vi "Event Handler.vi"(8 "error in":errorcluster, 10 "Stop Event Handler":refnum<user-event>, 11 "ScrollZoomGraphChart in":refnum<class "ScrollZoomGraphChart.lvclass">) -> (0 "error out":errorcluster)   [LabVIEW 2021, in "ScrollZoomGraphChart.lvclass"]
doc: "The <b>Event Handler VI</b> is a dynamic dispatch VI that should be overwritten if events are needed to create the enhanced QControl. \n\nBy inheriting from the main Control.lvclass the overwritten <b>Event Handler VI</b> will be launched asynchronously in the initialization of the QControl.\n<b> </b> <b> </b>\n©2016 Q Software Innovations, LLC (QSI)\nwritten by Quentin Alldredge\nproduced in LabVIEW 2015\n\nsupport@qsoftwareinnovations.com\nwww.qsoftwareinnovations.com\n\nAll rights reserved.\n\nRedistribution and use in source and binary forms, with or without modification, are permitted provided that the following conditions are met:\n\n * Redistributions of source code must retain the above copyright notice, this list of conditions and the following disclaimer.\n * Redistributions in binary form must reproduce the above copyright notice, this list of conditions and the following disclaimer in the documentation and/or other materials provided with the distribution.\n * Neither the name of Q Software Innovations, LLC. nor the names of its contributors may be used to endorse or promote products derived from this software without specific prior written permission.\n\nTHIS SOFTWARE IS PROVIDED BY THE COPYRIGHT HOLDERS AND CONTRIBUTORS \"AS IS\" AND ANY EXPRESS OR IMPLIED WARRANTIES, INCLUDING, BUT NOT LIMITED TO, THE IMPLIED WARRANTIES OF MERCHANTABILITY AND FITNESS FOR A PARTICULAR PURPOSE ARE DISCLAIMED. IN NO EVENT SHALL THE COPYRIGHT OWNER OR CONTRIBUTORS BE LIABLE FOR ANY DIRECT, INDIRECT, INCIDENTAL, SPECIAL, EXEMPLARY, OR CONSEQUENTIAL DAMAGES (INCLUDING, BUT NOT LIMITED TO, PROCUREMENT OF SUBSTITUTE GOODS OR SERVICES; LOSS OF USE, DATA, OR PROFITS; OR BUSINESS INTERRUPTION) HOWEVER CAUSED AND ON ANY THEORY OF LIABILITY, WHETHER IN CONTRACT, STRICT LIABILITY, OR TORT (INCLUDING NEGLIGENCE OR OTHERWISE) ARISING IN ANY WAY OUT OF THE USE OF THIS SOFTWARE, EVEN IF ADVISED OF THE POSSIBILITY OF SUCH DAMAGE."
uses:
  ScrollZoomGraphChart.lvclass
  ScrollZoomGraphChart.lvclass/ScrollZoomGraphChart.ctl
  <vilib>/Analysis/geometry.llb/Point in Polygon Position.ctl
  <vilib>/Analysis/NI_AAL_Geometry.lvlib
  c12e3cb6-15a2-4a40-9144-b1003a9e759b.vi
  c19ac079-acbd-42d5-82d2-a79b3126a602.vi
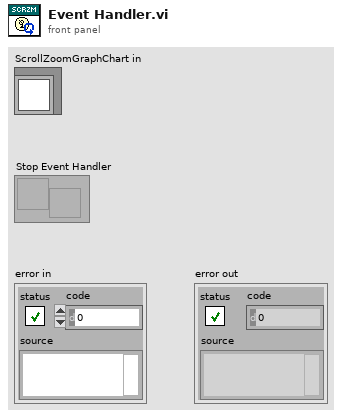
[diagram p1: front panel]
types:
  T1 = typedef "ScrollZoomGraphChart.lvclass/State Data.ctl" = cluster{"X Scales":refnum<vi>[], "Y Scales":refnum<vi>[], "Owning VI":refnum<vi>}
  T2 = typedef "NI_AAL_Geometry.lvlib/Point in Polygon Position.ctl" = u16
  T3 = typedef "LVPoint32TypeDef.ctl" = cluster{"Horizontal":i32, "Vertical":i32}
  T4 = cluster{"Shift":bool, "Ctrl":bool, "Alt":bool, "Cmd":bool, "Opt":bool}
  T5 = typedef "LVRectTypeDef.ctl" = cluster{"Left":i16, "Top":i16, "Right":i16, "Bottom":i16}
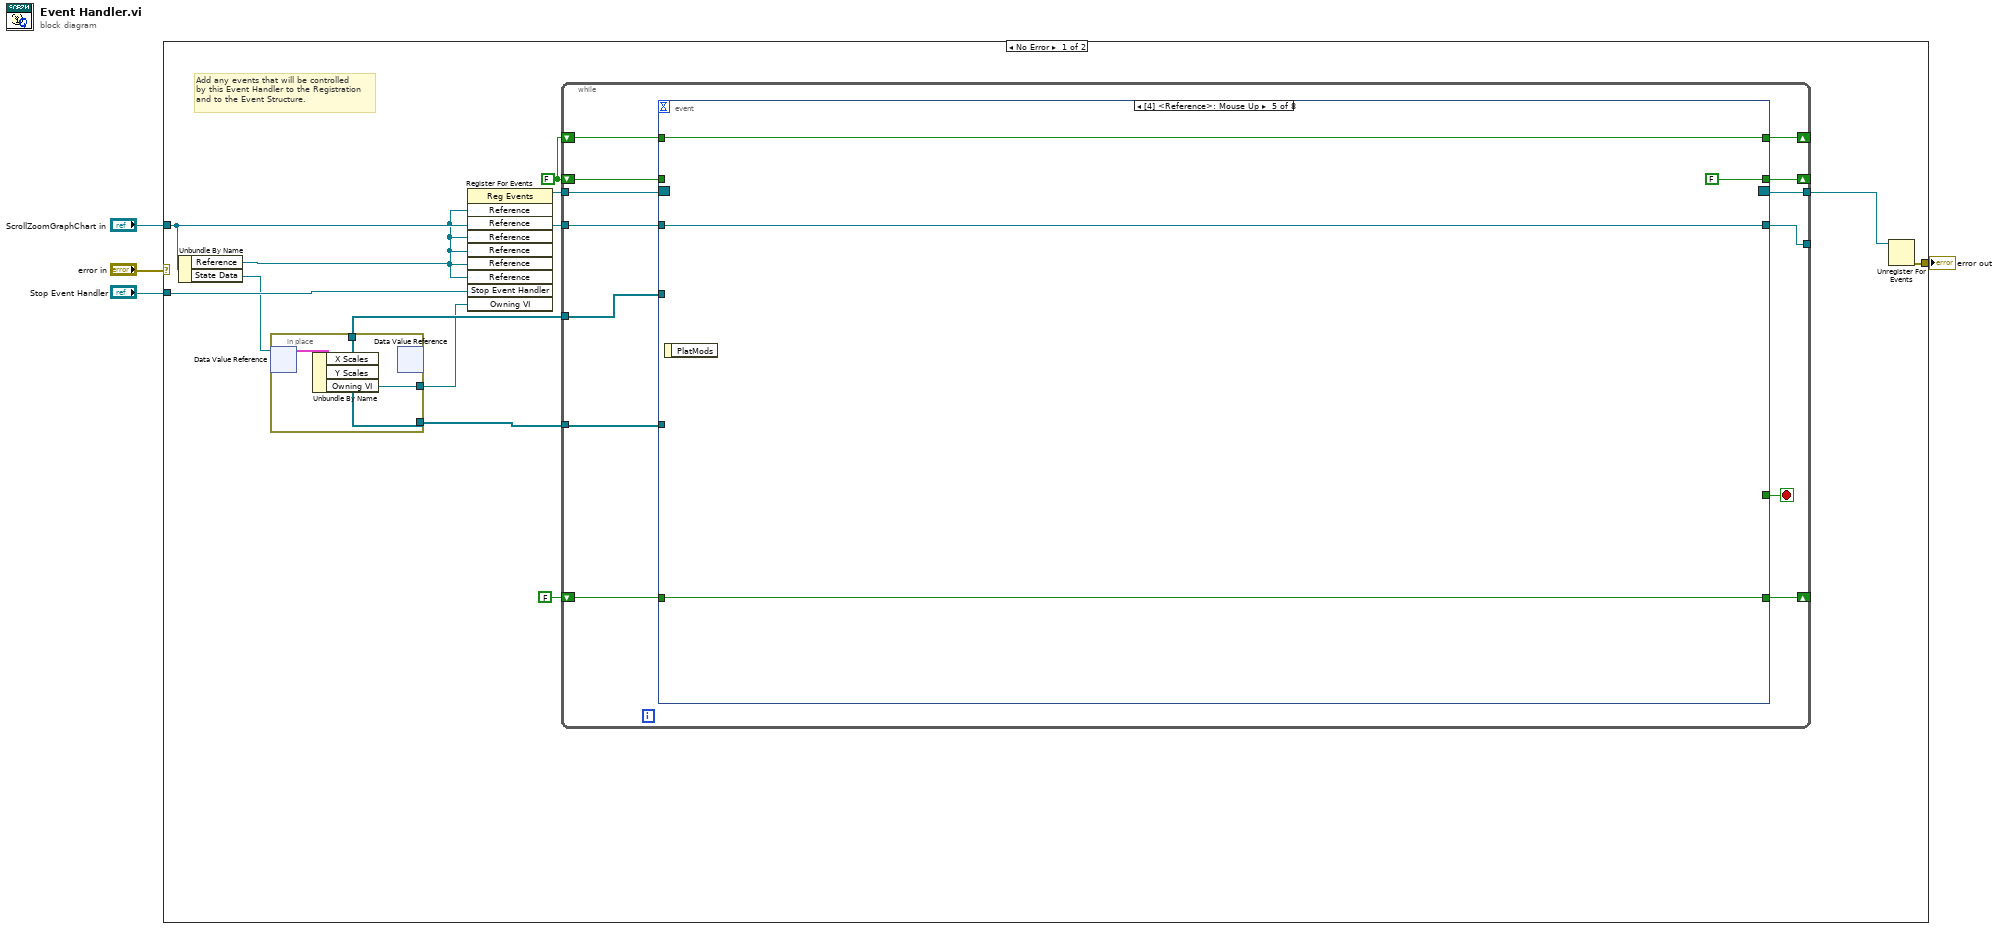
[diagram p0: block diagram]
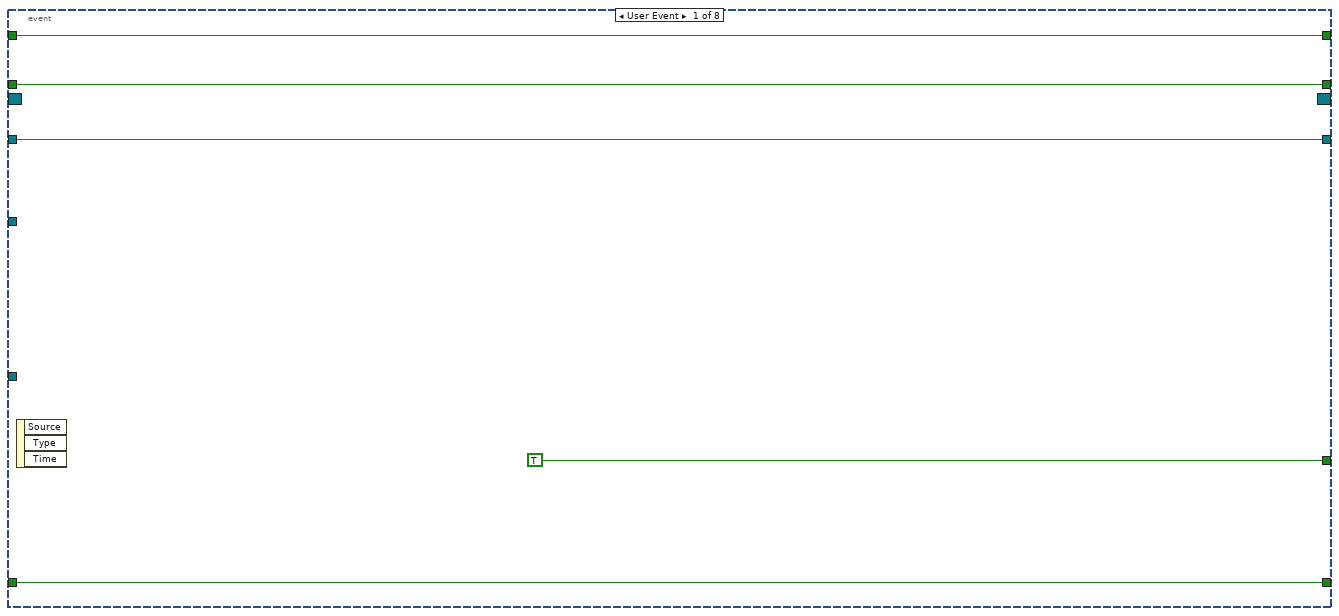
[diagram p2: hidden frame]
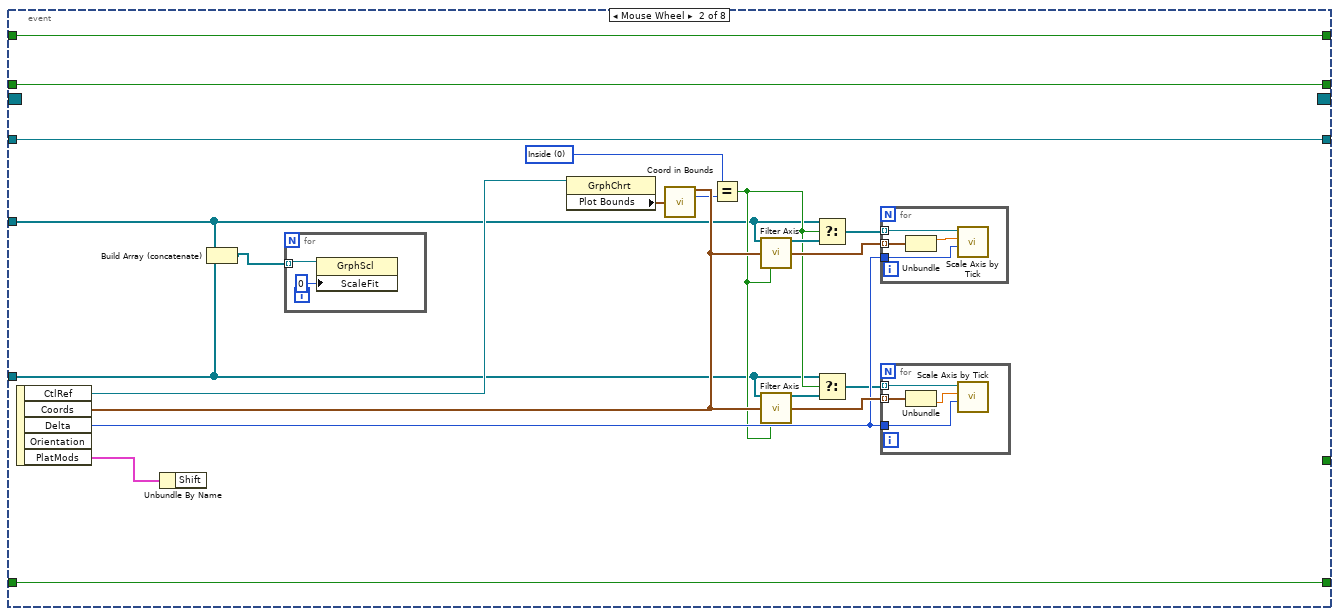
[diagram p3: hidden frame]
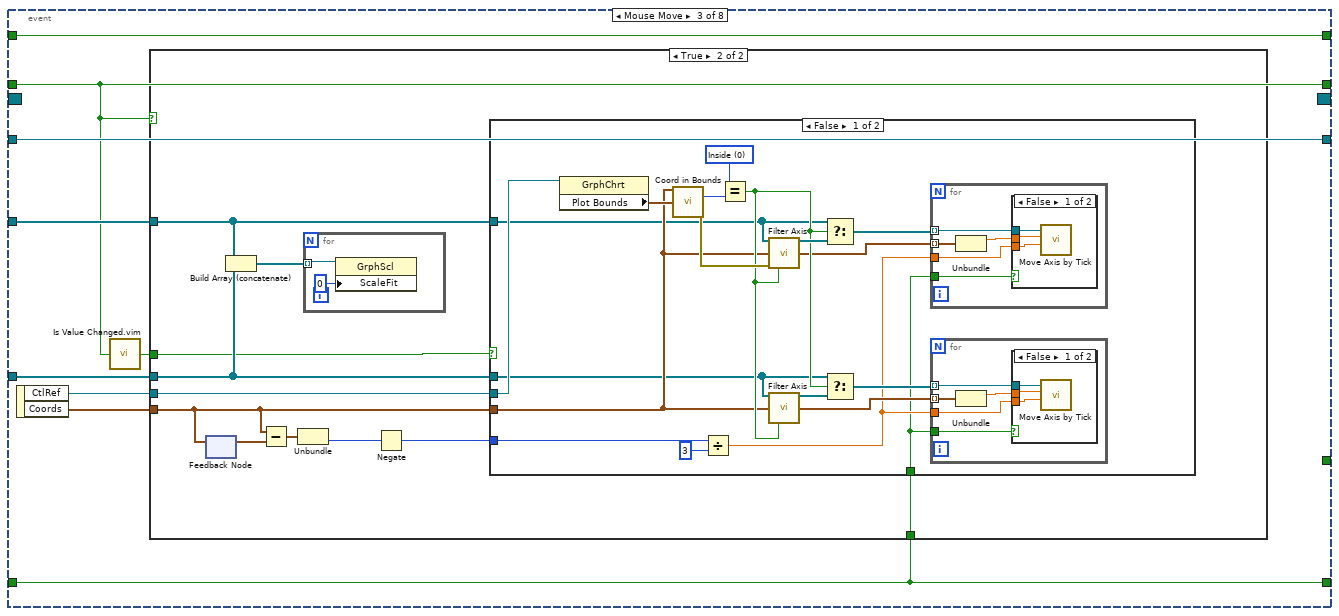
[diagram p4: hidden frame]
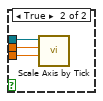
[diagram p6: hidden frame]
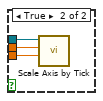
[diagram p7: hidden frame]
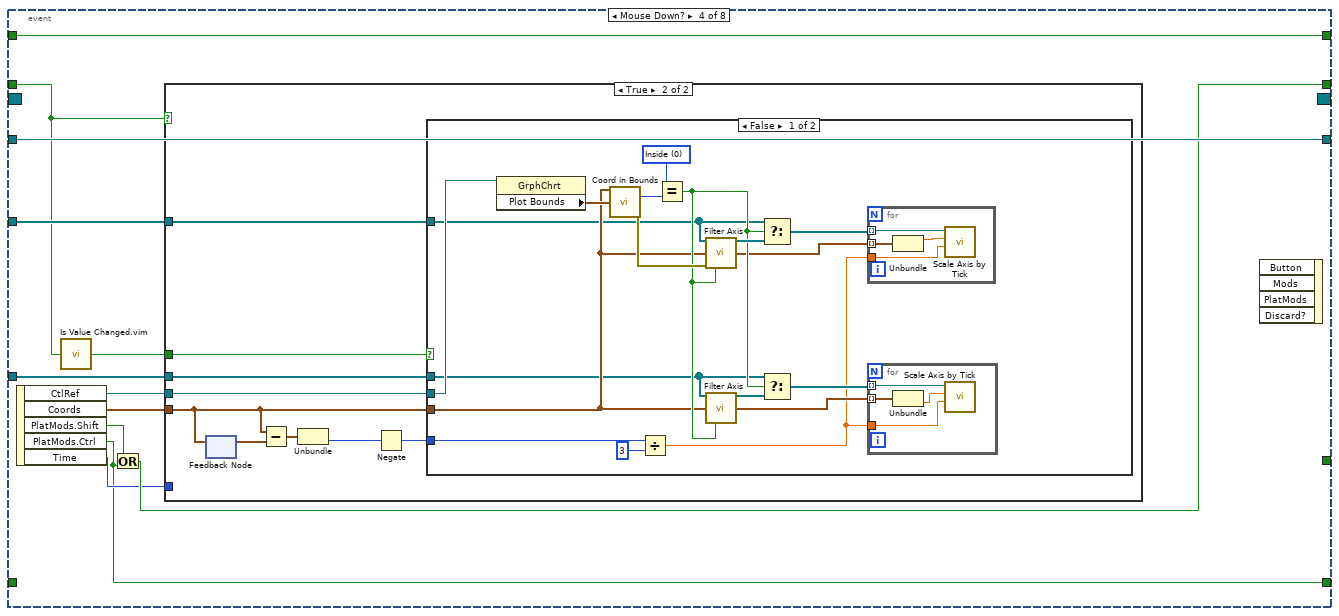
[diagram p9: hidden frame]
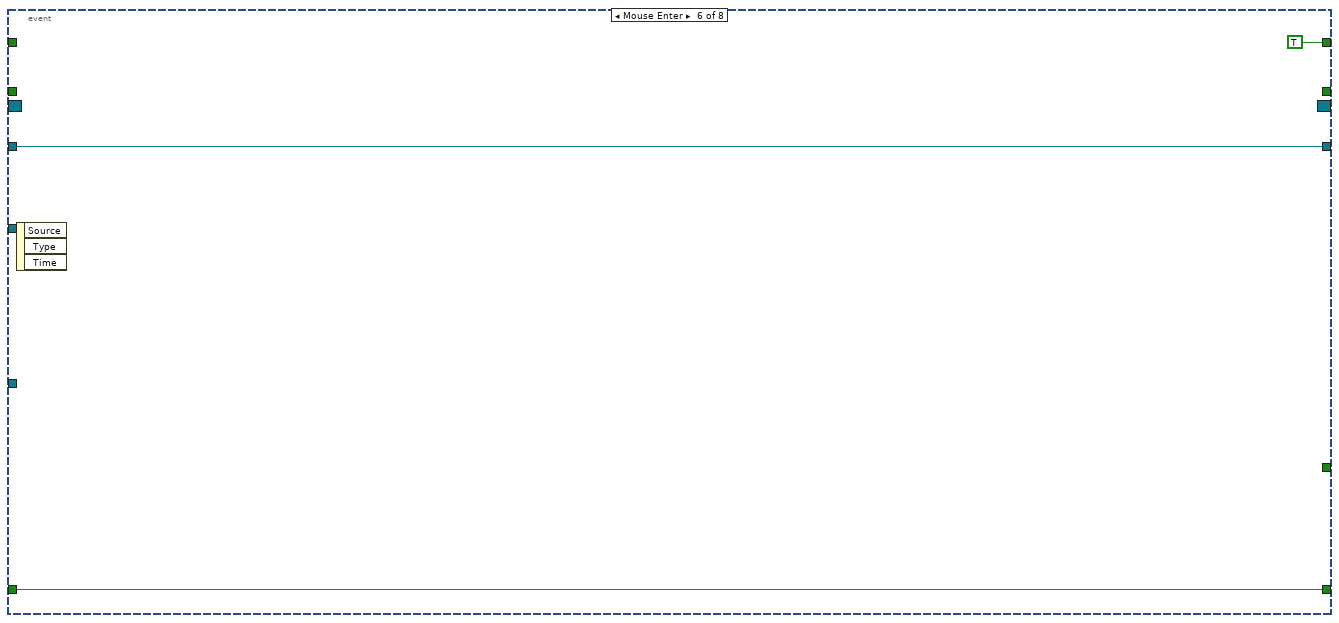
[diagram p12: hidden frame]
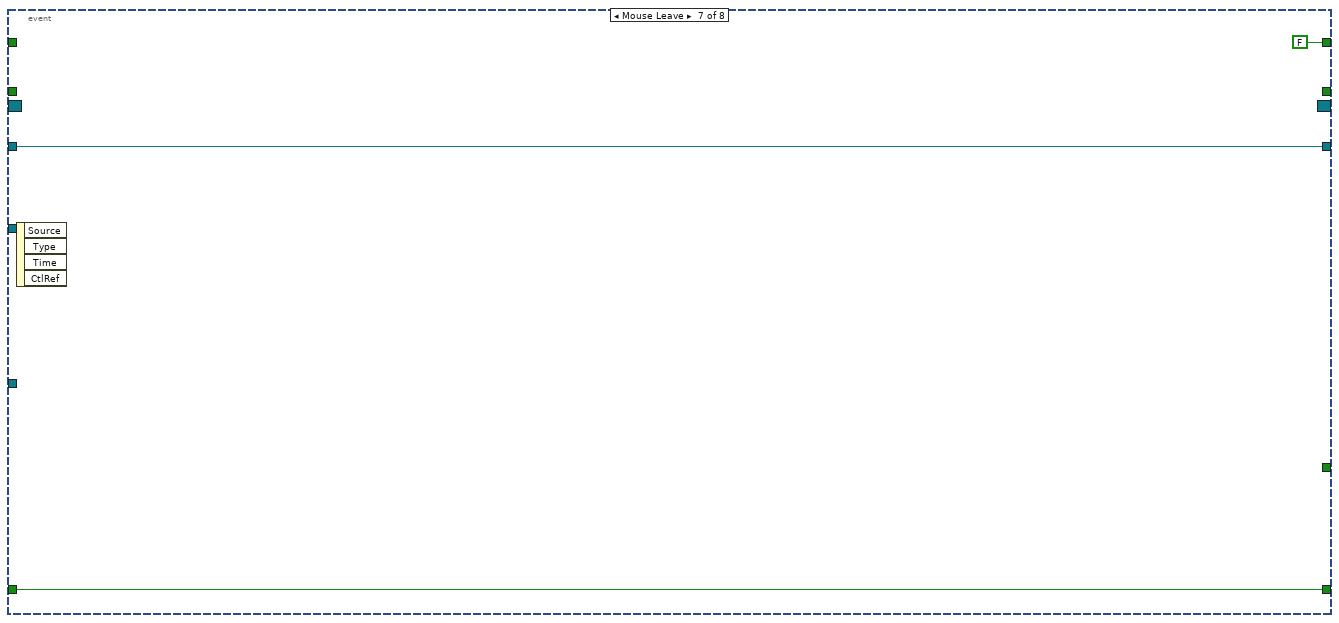
[diagram p13: hidden frame]
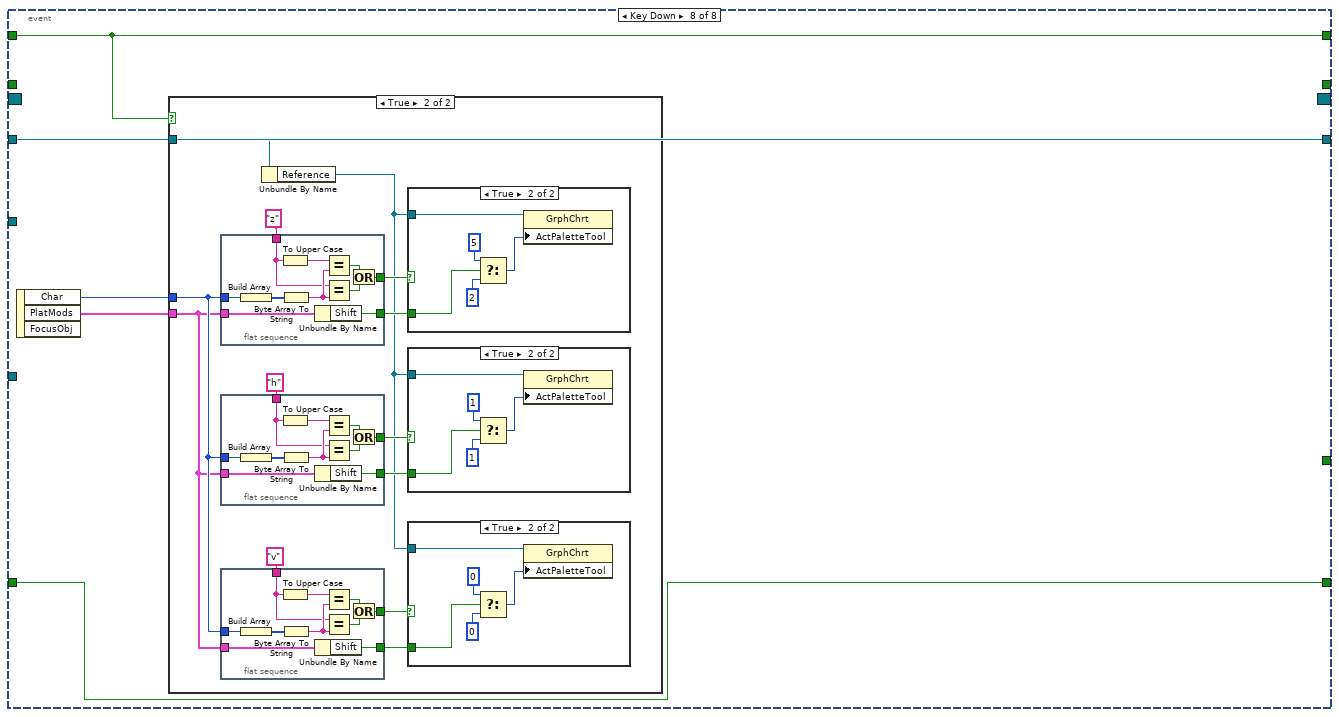
[diagram p14: hidden frame]
diagram:
  n1 = case shown="No Error" "error in" {
    selector: "error in" -> [_ w253]
    tunnel: [w16 w253] -> w3
    tunnel: "ScrollZoomGraphChart in" -> [w13 _]
    tunnel: "Stop Event Handler" -> [w15 _]
    frame No Error {
      w8 = FALSE
      # "Add any events that will be controlled\nby this Event Handler to the Registration\nand to the Event Structure."
      n2 = Unbundle By Name(w13) -> ("Reference"=w7:refnum<vi>, "State Data"=w12:refnum<data-value>)
      n3 = in-place {
        in-place-border: [w19] -> w11
        in-place-border: [w18] -> w10
        in-place-border: [w17] -> w5
        n4 = in-place-dvr #1(w12) -> (w20:T1)  [unwired: 1 out]
        n5 = Unbundle By Name(w20) -> ("X Scales"=w19:refnum<vi>[], "Y Scales"=w18:refnum<vi>[], "Owning VI"=w17:refnum<vi>)
        n6 = in-place-dvr #1() -> ()  [unwired: 1 in, 2 out]
      }
      n7 = register-events(w7, w7, w7, w7, w7, w7, w15, w5) -> (reference out=w14:refnum<event-registration>)  [unwired: 2 in, 1 out]
      n8 = while {
        tunnel: w11 -> [w32]
        tunnel: w10 -> [w31]
        tunnel: w14 -> [w30]
        tunnel: [w29] -> _
        tunnel: w13 -> [w28]
        tunnel: [w27] -> w9
        shift-right: [w26] -> _
        shift-left: w8 -> [w25]
        shift-right: [w23] -> _
        shift-left: w8 -> [w24]
        shift-right: [w22] -> _
        shift-left: FALSE ("Ctrl") -> [w21]
        stop <- w33 stop-if-true
        n9 = event shown="[4] <Reference>: Mouse Up" {
          selector: w30 -> [_ _ _ _ _ _ _ _]
          dyn-events: [_ _ _ _ _ _ _ _] -> w27
          timeout: _ -> [_ _ _ _ _ _ _ _]
          tunnel: [TRUE _ _ _ _ _ _ _] -> w33
          tunnel: w32 -> [_ w45 w77 w143 _ _ _ _]
          tunnel: w31 -> [_ w44 w76 w142 _ _ _ _]
          tunnel: [w36 w46 w78 w144 w182 w186 w189 w194] -> w29
          tunnel: w28 -> [w36 w46 w78 w144 w182 w186 w189 w194]
          tunnel: [w37 w42 w72 w138 FALSE _ _ _] -> w26
          tunnel: w25 -> [w37 w42 w72 w137 _ _ _ _]
          tunnel: w24 -> [w35 w41 w71 w135 w181 _ _ w191]
          tunnel: [w35 w41 w71 w135 w181 TRUE FALSE w191] -> w23
          tunnel: [w34 w39 w70 w133 w180 w184 w187 w190] -> w22
          tunnel: w21 -> [w34 w39 w70 _ w180 w184 w187 w190]
          event User Event {
            n10 = event-data() -> ()  [unwired: 1 in, 3 out]
          }
          event Mouse Wheel {
            w54 = T2 0 items=["Inside", "On Boundary", "Outside"] ("x")
            n11 = event-data() -> ("CtlRef"=w53:refnum<vi>, "Coords"=w56:T3, "Delta"=w50:i32, "PlatMods"=w40:T4)  [unwired: 1 in, 1 out]
            n12 = Unbundle By Name(w40) -> ()  [unwired: 1 out]
            n13 = Build Array (concatenate)(w45, w44) -> (w43:refnum<vi>[])
            n14 = for {
              tunnel: w43 -> [w61] mode=indexing
              n15 = property class="GrphScl"(reference=w61, "ScaleFit"=u8 0 ("Scale Fit")) -> ()  [unwired: 1 in, 2 out]
            }
            n16 = property class="GrphChrt"(reference=w53) -> ("Plot Bounds"=w57:T5)  [unwired: 1 in, 2 out]
            n17 = call "Coord in Bounds.vi"("Coords"=w56, "Plot Bounds"=w57) -> ("position"=w55:T2)  [unwired: 12 in, 1 out]
            n18 = Equal?(x=w54, y=w55) -> (x = y?=w47:bool)
            n19 = call "Filter Axis.vi"("Graph Scale in"=w45, "Coords"=w56, "Bypass Filter"=w47) -> ("Filter Graph Scale out"=w59:refnum<vi>[], "Axis Value"=w58:cluster{"X":dbl, "Y":dbl}[])  [unwired: 10 in, 1 out]
            n20 = call "Filter Axis.vi"("Graph Scale in"=w44, "Coords"=w56, "Bypass Filter"=w47) -> ("Filter Graph Scale out"=w52:refnum<vi>[], "Axis Value"=w51:cluster{"X":dbl, "Y":dbl}[])  [unwired: 10 in, 1 out]
            n21 = Select(t=w45, s=w47, f=w59) -> (s? t:f=w49:refnum<vi>[])
            n22 = Select(t=w44, s=w47, f=w52) -> (s? t:f=w48:refnum<vi>[])
            n23 = for {
              tunnel: w49 -> [w69] mode=indexing
              tunnel: w58 -> [w68] mode=indexing
              tunnel: w50 -> [w66]
              n24 = Unbundle(w68) -> ("X"=w67:dbl)  [unwired: 1 out]
              n25 = call "Scale Axis by Tick.vi"("Tick Scale"=w66, "Axis Focus Value"=w67, "GraphScale in"=w69) -> ()  [unwired: 9 in]
            }
            n26 = for {
              tunnel: w48 -> [w65] mode=indexing
              tunnel: w51 -> [w64] mode=indexing
              tunnel: w50 -> [w63]
              n27 = Unbundle(w64) -> ("Y"=w62:dbl)  [unwired: 1 out]
              n28 = call "Scale Axis by Tick.vi"("Tick Scale"=w63, "Axis Focus Value"=w62, "GraphScale in"=w65) -> ()  [unwired: 9 in]
            }
          }
          event Mouse Move {
            n29 = event-data() -> ("CtlRef"=w74:refnum<vi>, "Coords"=w73:T3)  [unwired: 1 in]
            n30 = call "Is Value Changed.vim"("value"=w72) -> ("changed or first call?"=w75:bool)
            n31 = case shown="True" w72 {
              tunnel: w73 -> [_ w85]
              tunnel: w74 -> [_ w89]
              tunnel: w77 -> [_ w88]
              tunnel: w76 -> [_ w87]
              tunnel: w75 -> [_ w82]
              tunnel: w70 -> [_ w79]
              frame False {
              }
              frame True {
                n32 = feedback-in #2(w85) -> ()
                n33 = feedback #2() -> (w84:T3)  [unwired: 1 in]
                n34 = Build Array (concatenate)(w88, w87) -> (w86:refnum<vi>[])
                n35 = Subtract(x=w85, y=w84) -> (x-y=w83:T3)
                n36 = Unbundle(w83) -> ("Vertical"=w81:i32)  [unwired: 1 out]
                n37 = for {
                  tunnel: w86 -> [w91] mode=indexing
                  n38 = property class="GrphScl"(reference=w91, "ScaleFit"=u8 0 ("Scale Fit")) -> ()  [unwired: 1 in, 2 out]
                }
                n39 = Negate(x=w81) -> (-x=w80:i32)
                n40 = case shown="False" w82 {
                  tunnel: w89 -> [w108 _]
                  tunnel: w88 -> [w97 _]
                  tunnel: w87 -> [w96 _]
                  tunnel: w85 -> [w101 _]
                  tunnel: w80 -> [w104 _]
                  tunnel: w79 -> [w92 _]
                  frame False {
                    w100 = T2 0 items=["Inside", "On Boundary", "Outside"] ("x")
                    n41 = property class="GrphChrt"(reference=w108) -> ("Plot Bounds"=w102:T5)  [unwired: 1 in, 2 out]
                    n42 = call "Coord in Bounds.vi"("Coords"=w101, "Plot Bounds"=w102) -> ("position"=w99:T2, "error out"=w110:errorcluster)  [unwired: 12 in]
                    n43 = Divide(x=w104, y=3) -> (x/y=w93:dbl)
                    n44 = Equal?(x=w100, y=w99) -> (x = y?=w105:bool)
                    n45 = call "Filter Axis.vi"("Graph Scale in"=w97, "Coords"=w101, "error in"=w110, "Bypass Filter"=w105) -> ("Filter Graph Scale out"=w109:refnum<vi>[], "Axis Value"=w98:cluster{"X":dbl, "Y":dbl}[])  [unwired: 9 in, 1 out]
                    n46 = call "Filter Axis.vi"("Graph Scale in"=w96, "Coords"=w101, "Bypass Filter"=w105) -> ("Filter Graph Scale out"=w107:refnum<vi>[], "Axis Value"=w94:cluster{"X":dbl, "Y":dbl}[])  [unwired: 10 in, 1 out]
                    n47 = Select(t=w97, s=w105, f=w109) -> (s? t:f=w106:refnum<vi>[])
                    n48 = Select(t=w96, s=w105, f=w107) -> (s? t:f=w95:refnum<vi>[])
                    n49 = for {
                      tunnel: w106 -> [w126] mode=indexing
                      tunnel: w98 -> [w125] mode=indexing
                      tunnel: w93 -> [w124]
                      tunnel: w92 -> [w122]
                      n50 = Unbundle(w125) -> ("X"=w123:dbl)  [unwired: 1 out]
                      n51 = case shown="False" w122 {
                        tunnel: w126 -> [w129 w132]
                        tunnel: w124 -> [w127 w131]
                        tunnel: w123 -> [w128 w130]
                        frame False {
                          n52 = call "Move Axis by Tick.vi"("Tick Scale"=w127, "Axis Focus Value"=w128, "GraphScale in"=w129) -> ()  [unwired: 9 in]
                        }
                        frame True {
                          n53 = call "Scale Axis by Tick.vi"("Tick Scale"=w131, "Axis Focus Value"=w130, "GraphScale in"=w132) -> ()  [unwired: 9 in]
                        }
                      }
                    }
                    n54 = for {
                      tunnel: w95 -> [w115] mode=indexing
                      tunnel: w94 -> [w114] mode=indexing
                      tunnel: w93 -> [w113]
                      tunnel: w92 -> [w111]
                      n55 = Unbundle(w114) -> ("X"=w112:dbl)  [unwired: 1 out]
                      n56 = case shown="False" w111 {
                        tunnel: w115 -> [w118 w121]
                        tunnel: w113 -> [w116 w120]
                        tunnel: w112 -> [w117 w119]
                        frame False {
                          n57 = call "Move Axis by Tick.vi"("Tick Scale"=w116, "Axis Focus Value"=w117, "GraphScale in"=w118) -> ()  [unwired: 9 in]
                        }
                        frame True {
                          n58 = call "Scale Axis by Tick.vi"("Tick Scale"=w120, "Axis Focus Value"=w119, "GraphScale in"=w121) -> ()  [unwired: 9 in]
                        }
                      }
                    }
                  }
                  frame True {
                  }
                }
              }
            }
          }
          event Mouse Down? {
            n59 = event-data() -> ("CtlRef"=w140:refnum<vi>, "Coords"=w139:T3, "PlatMods.Shift"=w136:bool, "PlatMods.Ctrl"=w133:bool, "Time"=w134:u32)  [unwired: 1 in]
            n60 = call "Is Value Changed.vim"("value"=w137) -> ("changed or first call?"=w141:bool)
            n61 = Or(x=w136, y=w133) -> (x .or. y?=w138:bool)
            n62 = case shown="True" w137 {
              tunnel: w139 -> [_ w150]
              tunnel: w140 -> [_ w153]
              tunnel: w143 -> [_ w152]
              tunnel: w142 -> [_ w151]
              tunnel: w141 -> [_ w147]
              tunnel: w134 -> [_ _]
              frame False {
              }
              frame True {
                n63 = feedback-in #3(w150) -> ()
                n64 = feedback #3() -> (w149:T3)  [unwired: 1 in]
                n65 = Subtract(x=w150, y=w149) -> (x-y=w148:T3)
                n66 = Unbundle(w148) -> ("Vertical"=w146:i32)  [unwired: 1 out]
                n67 = Negate(x=w146) -> (-x=w145:i32)
                n68 = case shown="False" w147 {
                  tunnel: w153 -> [w169 _]
                  tunnel: w152 -> [w155 _]
                  tunnel: w151 -> [w154 _]
                  tunnel: w150 -> [w159 _]
                  tunnel: w145 -> [w163 _]
                  frame False {
                    w158 = T2 0 items=["Inside", "On Boundary", "Outside"] ("x")
                    n69 = property class="GrphChrt"(reference=w169) -> ("Plot Bounds"=w160:T5)  [unwired: 1 in, 2 out]
                    n70 = call "Coord in Bounds.vi"("Coords"=w159, "Plot Bounds"=w160) -> ("position"=w157:T2, "error out"=w171:errorcluster)  [unwired: 12 in]
                    n71 = Divide(x=w163, y=3) -> (x/y=w161:dbl)
                    n72 = Equal?(x=w158, y=w157) -> (x = y?=w164:bool)
                    n73 = call "Filter Axis.vi"("Graph Scale in"=w155, "Coords"=w159, "error in"=w171, "Bypass Filter"=w164) -> ("Filter Graph Scale out"=w170:refnum<vi>[], "Axis Value"=w156:cluster{"X":dbl, "Y":dbl}[])  [unwired: 9 in, 1 out]
                    n74 = call "Filter Axis.vi"("Graph Scale in"=w154, "Coords"=w159, "Bypass Filter"=w164) -> ("Filter Graph Scale out"=w168:refnum<vi>[], "Axis Value"=w167:cluster{"X":dbl, "Y":dbl}[])  [unwired: 10 in, 1 out]
                    n75 = Select(t=w155, s=w164, f=w170) -> (s? t:f=w166:refnum<vi>[])
                    n76 = Select(t=w154, s=w164, f=w168) -> (s? t:f=w165:refnum<vi>[])
                    n77 = for {
                      tunnel: w166 -> [w179] mode=indexing
                      tunnel: w156 -> [w178] mode=indexing
                      tunnel: w161 -> [w177]
                      n78 = Unbundle(w178) -> ("X"=w176:dbl)  [unwired: 1 out]
                      n79 = call "Scale Axis by Tick.vi"("Tick Scale"=w177, "Axis Focus Value"=w176, "GraphScale in"=w179) -> ()  [unwired: 9 in]
                    }
                    n80 = for {
                      tunnel: w165 -> [w175] mode=indexing
                      tunnel: w167 -> [w174] mode=indexing
                      tunnel: w161 -> [w173]
                      n81 = Unbundle(w174) -> ("Y"=w172:dbl)  [unwired: 1 out]
                      n82 = call "Scale Axis by Tick.vi"("Tick Scale"=w173, "Axis Focus Value"=w172, "GraphScale in"=w175) -> ()  [unwired: 9 in]
                    }
                  }
                  frame True {
                  }
                }
              }
            }
            n83 = event-data() -> ()  [unwired: 5 in, 1 out]
          }
          event Mouse Up {
            n84 = event-data() -> ()  [unwired: 1 in, 1 out]
          }
          event Mouse Enter {
            n85 = event-data() -> ()  [unwired: 1 in, 3 out]
          }
          event Mouse Leave {
            n86 = event-data() -> ()  [unwired: 1 in, 4 out]
          }
          event Key Down {
            n87 = event-data() -> ("Char"=w193:i16, "PlatMods"=w192:T4)  [unwired: 1 in, 1 out]
            n88 = case shown="True" w191 {
              tunnel: w194 -> [_ w207]
              tunnel: w193 -> [_ w200]
              tunnel: w192 -> [_ w199]
              frame False {
              }
              frame True {
                n89 = flat-sequence {
                  tunnel: w200 -> [w247]
                  tunnel: [w241] -> w206
                  tunnel: w199 -> [w240]
                  tunnel: [w239] -> w205
                  tunnel: "z" -> [w238]
                  frame #0 {
                    n90 = Build Array(w247) -> (w246:i16[])
                    n91 = To Upper Case(1:w238) -> (0:w245:string)
                    n92 = Byte Array To String(unsigned byte array=w246) -> (string=w244:string)
                    n93 = Unbundle By Name(w240) -> ("Shift"=w239:bool)
                    n94 = Equal?(x=w245, y=w244) -> (x = y?=w243:bool)
                    n95 = Equal?(x=w238, y=w244) -> (x = y?=w242:bool)
                    n96 = Or(x=w243, y=w242) -> (x .or. y?=w241:bool)
                  }
                }
                n97 = flat-sequence {
                  tunnel: w200 -> [w237]
                  tunnel: [w231] -> w202
                  tunnel: w199 -> [w230]
                  tunnel: [w229] -> w201
                  tunnel: "h" -> [w228]
                  frame #0 {
                    n98 = Build Array(w237) -> (w236:i16[])
                    n99 = To Upper Case(1:w228) -> (0:w235:string)
                    n100 = Byte Array To String(unsigned byte array=w236) -> (string=w234:string)
                    n101 = Unbundle By Name(w230) -> ("Shift"=w229:bool)
                    n102 = Equal?(x=w235, y=w234) -> (x = y?=w233:bool)
                    n103 = Equal?(x=w228, y=w234) -> (x = y?=w232:bool)
                    n104 = Or(x=w233, y=w232) -> (x .or. y?=w231:bool)
                  }
                }
                n105 = flat-sequence {
                  tunnel: w200 -> [w222]
                  tunnel: [w216] -> w196
                  tunnel: w199 -> [w215]
                  tunnel: [w214] -> w195
                  tunnel: "v" -> [w213]
                  frame #0 {
                    n106 = Build Array(w222) -> (w221:i16[])
                    n107 = To Upper Case(1:w213) -> (0:w220:string)
                    n108 = Byte Array To String(unsigned byte array=w221) -> (string=w219:string)
                    n109 = Unbundle By Name(w215) -> ("Shift"=w214:bool)
                    n110 = Equal?(x=w220, y=w219) -> (x = y?=w218:bool)
                    n111 = Equal?(x=w213, y=w219) -> (x = y?=w217:bool)
                    n112 = Or(x=w218, y=w217) -> (x .or. y?=w216:bool)
                  }
                }
                n113 = Unbundle By Name(w207) -> ("Reference"=w197:refnum<vi>)
                n114 = case shown="True" w206 {
                  tunnel: w197 -> [_ w252]
                  tunnel: w205 -> [_ w251]
                  frame False {
                  }
                  frame True {
                    n115 = Select(t=5 ("Palette:Active Tool"), s=w251, f=2) -> (s? t:f=w248:i32)
                    n116 = property class="GrphChrt"(reference=w252, "ActPaletteTool"=w248) -> ()  [unwired: 1 in, 2 out]
                  }
                }
                n117 = case shown="True" w202 {
                  tunnel: w197 -> [_ w227]
                  tunnel: w201 -> [_ w226]
                  frame False {
                  }
                  frame True {
                    n118 = Select(t=1 ("Palette:Active Tool"), s=w226, f=1) -> (s? t:f=w223:i32)
                    n119 = property class="GrphChrt"(reference=w227, "ActPaletteTool"=w223) -> ()  [unwired: 1 in, 2 out]
                  }
                }
                n120 = case shown="True" w196 {
                  tunnel: w197 -> [_ w212]
                  tunnel: w195 -> [_ w211]
                  frame False {
                  }
                  frame True {
                    n121 = Select(t=0 ("Palette:Active Tool"), s=w211, f=0) -> (s? t:f=w208:i32)
                    n122 = property class="GrphChrt"(reference=w212, "ActPaletteTool"=w208) -> ()  [unwired: 1 in, 2 out]
                  }
                }
              }
            }
          }
        }
      }
      n123 = Unregister For Events(event registration refnum=w9) -> (error out=w16:errorcluster)  [unwired: 1 in]
    }
    frame Error {
    }
  }
  "error out" <- w3
